vi "yaqc_in_limits.vi"(7 "Position":dbl, 8 "error in (no error)":errorcluster, 9 "Yaqc Client In":refnum<k38>, 10 "Python Module Path In":path, 11 "Python Session In":refnum<k35>) -> (0 "error out":errorcluster, 1 "Yaqc Client Out":refnum<k38>, 2 "Python Module Path Out":path, 3 "Python Session Out":refnum<k35>, 4 "InLimits?":bool)   [LabVIEW 2022 SP3]
doc: "Determines if a value supplied is within the limits of the device."
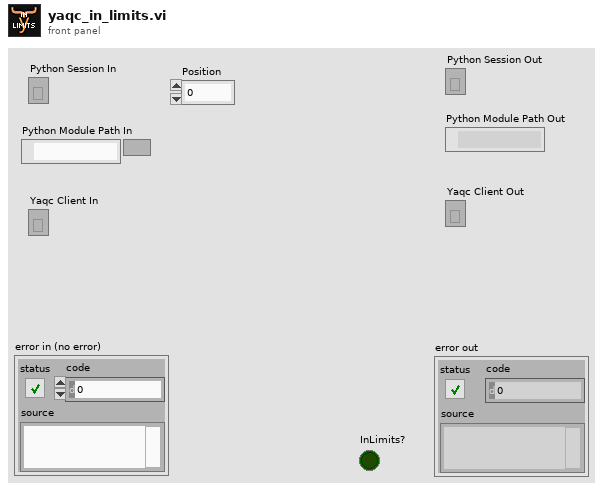
[diagram p1: front panel]
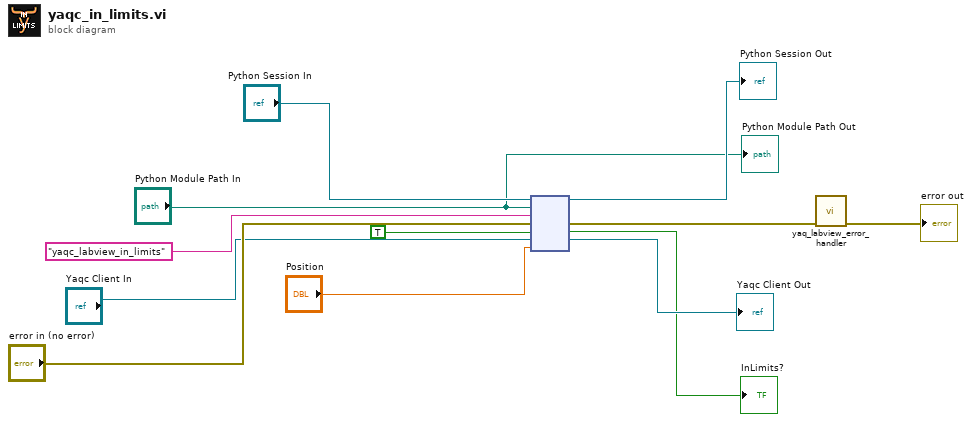
[diagram p0: block diagram]
diagram:
  n1 = node("Python Session In", "Python Module Path In", "yaqc_labview_in_limits" ("function name"), "error in (no error)", TRUE, "Yaqc Client In", "Position") -> (→"Python Session Out":refnum<k35>, w9:errorcluster, →"InLimits?":bool, →"Yaqc Client Out":refnum<k38>)  [unwired: 1 in, 2 out]
  n2 = call "yaq_labview_error_handler.vi"("error in (no error)"=w9) -> ("error out"=→"error out":errorcluster)  [unwired: 10 in]
  "Python Module Path Out" <- "Python Module Path In"
